vi "Translation3d_Div.vi"(9 "Scalar":dbl, 11 "In Translation3d":T1 {"Z" format="%14.3f"; "Y" format="%14.3f"; "X" format="%14.3f"}) -> (3 "Out Translation3d":T1 {"Z" format="%14.3f"; "Y" format="%14.3f"; "X" format="%14.3f"})   [LabVIEW 2019, in "Trajectory_Library.lvlib"]
doc: "Returns the translation divided by a scalar.\n \nFor example, Translation3d(2.0, 2.5, 4.5) / 2 = Translation3d(1.0, 1.25, 2.25).\n\nParameters:\n - In Translation3d - This translation3d data structure\n - scalar - The value to divide the translation by\n\nResult:\n - Out Translation3d - The resulting translation"
uses:
  Trajectory_Library.lvlib
  TypeDef/TRANSLATION3D.ctl
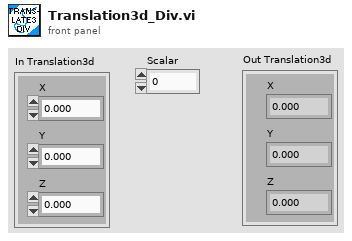
[diagram p1: front panel]
types:
  T1 = typedef "Trajectory_Library.lvlib/TRANSLATION3D.ctl" = cluster{"X":dbl, "Y":dbl, "Z":dbl}
  T2 = typedef "WPILib_Math.lvlib/TRANSLATION3D.ctl" = cluster{"X":dbl, "Y":dbl, "Z":dbl}
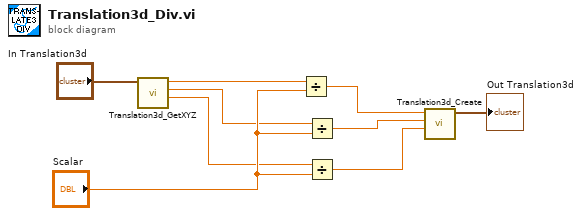
[diagram p0: block diagram]
diagram:
  n1 = call "Translation3d_GetXYZ.vi"("In Translation3d"="In Translation3d") -> ("Z"=w1:dbl, "Y"=w2:dbl, "X"=w3:dbl)  [unwired: 8 in]
  n2 = Divide(x=w3, y="Scalar") -> (x/y=w8:dbl)
  n3 = Divide(x=w2, y="Scalar") -> (x/y=w7:dbl)
  n4 = Divide(x=w1, y="Scalar") -> (x/y=w5:dbl)
  n5 = call "Translation3d_Create.vi"("Z"=w5, "Y"=w7, "X"=w8) -> ("TRANSLATION3D"=→"Out Translation3d":T2)  [unwired: 8 in]
